vi "Autotest.vi"(8 "error in (no error)":errorcluster caption="entrée d'erreur (pas d'erreur)", 11 "Class UART Nodon.lvclass En entrée":refnum<class "Class UART Nodon.lvclass">) -> (0 "error out":errorcluster caption="sortie d'erreur", 2 "Autotest Ok":bool, 3 "Class UART Nodon.lvclass En sortie":refnum<class "Class UART Nodon.lvclass">)   [LabVIEW 2020, in "Library Instrument & Equipement.lvlib" / "Library UART.lvlib" / "Class UART Nodon.lvclass"]
uses:
  Class UART Nodon.lvclass
  C:/Users/ngarcin/OneDrive - Altyor/Standard TB/Class/UART/UART (Default)/Class UART (Default).lvclass
  <vilib>/Instr/_visa.llb/VISA Find Search Mode.ctl
  UART (Default)/Class UART (Default).lvclass
  Class UART Nodon.lvclass/Class UART Nodon.ctl
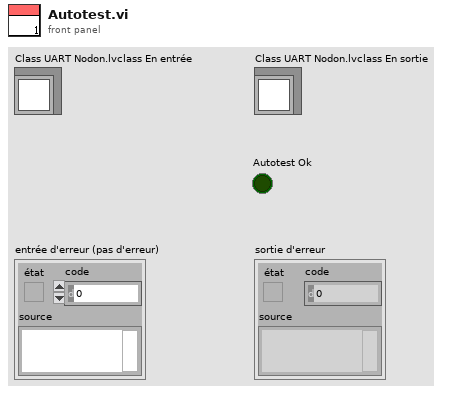
[diagram p1: front panel]
types:
  T1 = typedef "VISA Find Search Mode.ctl" = u32
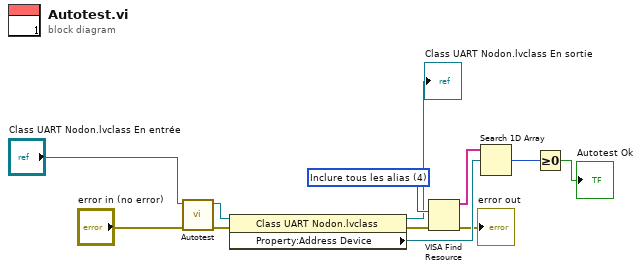
[diagram p0: block diagram]
diagram:
  w9 = T1 4 items=["Noms canoniques uniquement"=0, "Alias uniquement"=2, "Inclure les alias correspondants"=3, "Inclure tous les alias"=4] ("Search Mode")
  n1 = call-parent "Autotest.vi"("error in (no error)"="error in (no error)", "Class UART (Default) en entrée"="Class UART Nodon.lvclass En entrée") -> ("error out"=w3:errorcluster, "Class UART (Default) en sortie"=w5:refnum<class "Class UART Nodon.lvclass">)  [unwired: 7 in, 1 out]
  n2 = property class="Class UART Nodon.lvclass"(reference=w5, error in=w3) -> (reference out=→"Class UART Nodon.lvclass En sortie":refnum<class "Class UART Nodon.lvclass">, error out=w10:errorcluster, "Property:Address Device"=w8:refnum<visa-resource-name>)
  n3 = VISA Find Resource(8:w10, 10:w9) -> (0:→"error out":errorcluster, 3:w7:string[])  [unwired: 1 in, 1 out]
  n4 = Search 1D Array(1D array=w7, element=w8) -> (index of element=w6:i32)  [unwired: 1 in]
  n5 = Greater Or Equal To 0?(x=w6) -> (x >= 0?=→"Autotest Ok":bool)
